vi "CalGas Filtern für Endpunktkalibrieren.vi"(10 "Messbereich":u16, 11 "CalGas":u16) -> (0 "Einheit":T4, 1 "Messberich":T4, 2 "Wert 2":T11 format="%#_5g", 3 "Wert 1":T11 format="%#_5g", 4 "Fehler":bool, 5 "Name":T4, 6 "Array":T1[](array[typedef]) format="%#_5g", 7 "Messbereich":u16)   [LabVIEW 2020, in "CalGas Aufschaltung.lvlib"]
uses:
  CalGas Aufschaltung.lvlib
  Visualisierungs Elemente/Zahlen-Ausgabefeld.ctl
  Visualisierungs Elemente/String - Ausgabefeld.ctl
  Definition CalGas Anzeige.ctl
  CalGas-Namen.ctl
  Visualisierungs Elemente/String - Eingabefeld.ctl
  CalGas-Werte.ctl
  Visualisierungs Elemente/Zahlen-Eingabefeld.ctl
  CalGas-Einheit.ctl
  Visualisierungs Elemente/Auswahlfeld.ctl
  CalGas-Messbereiche.ctl
  Aufschaltung CalGas_ANZEIGE.ctl
  FGV CalGas Aktionen.ctl
panel:
  in  "Aufschaltung CalGas":T2 {"Analysator" items=["FT-IR"]; "Aufschaltpunkt" items=["über Filterblock", "Analysator direkt", "über Gasteiler"]; "Kalibriergas" items=["Stickstoff", "", "", "", "", "", "", "", "", "", "", "", ""]}
  in  "Def.CalGas":T5 {"Messbereiche"."Messbereich 12" items=["0-100ppm", "0-1000ppm", "0-5000ppm"]; "Messbereiche"."Messbereich 11" items=["0-100ppm", "0-1000ppm", "0-5000ppm"]; "Messbereiche"."Messbereich 10" items=["0-100ppm", "0-1000ppm", "0-5000ppm"]; "Messbereiche"."Messbereich 9" items=["0-100ppm", "0-1000ppm", "0-5000ppm"]; "Messbereiche"."Messbereich 8" items=["0-100ppm", "0-1000ppm", "0-5000ppm"]; "Messbereiche"."Messbereich 7" items=["0-100ppm", "0-1000ppm", "0-5000ppm"]; "Messbereiche"."Messbereich 6" items=["0-100ppm", "0-1000ppm", "0-5000ppm"]; "Messbereiche"."Messbereich 5" items=["0-100ppm", "0-1000ppm", "0-5000ppm"]; "Messbereiche"."Messbereich 4" items=["0-100ppm", "0-1000ppm", "0-5000ppm"]; "Messbereiche"."Messbereich 3" items=["0-100ppm", "0-1000ppm", "0-5000ppm"]; "Messbereiche"."Messbereich 2" items=["0-100ppm", "0-1000ppm", "0-5000ppm"]; "Messbereiche"."Messbereich 1" items=["0-100ppm", "0-1000ppm", "0-5000ppm"]; "Einheit"."Einheit 12" items=["ppm", "%"]; "Einheit"."Einheit 11" items=["ppm", "%"]; "Einheit"."Einheit 10" items=["ppm", "%"]; "Einheit"."Einheit 9" items=["ppm", "%"]; "Einheit"."Einheit 8" items=["ppm", "%"]; "Einheit"."Einheit 7" items=["ppm", "%"]; "Einheit"."Einheit 6" items=["ppm", "%"]; "Einheit"."Einheit 5" items=["ppm", "%"]; "Einheit"."Einheit 4" items=["ppm", "%"]; "Einheit"."Einheit 3" items=["ppm", "%"]; "Einheit"."Einheit 2" items=["ppm", "%"]; "Einheit"."Einheit 1" items=["ppm", "%"]; "Werte 2"."Konzentration 12" format="%#_5g"; "Werte 2"."Konzentration 11" format="%#_5g"; "Werte 2"."Konzentration 10" format="%#_5g"; "Werte 2"."Konzentration 9" format="%#_5g"; "Werte 2"."Konzentration 8" format="%#_5g"; "Werte 2"."Konzentration 7" format="%#_5g"; "Werte 2"."Konzentration 6" format="%#_5g"; "Werte 2"."Konzentration 5" format="%#_5g"; "Werte 2"."Konzentration 4" format="%#_5g"; "Werte 2"."Konzentration 3" format="%#_5g"; "Werte 2"."Konzentration 2" format="%#_5g"; "Werte 2"."Konzentration 1" format="%#_5g"; "Werte"."Konzentration 12" format="%#_5g"; "Werte"."Konzentration 11" format="%#_5g"; "Werte"."Konzentration 10" format="%#_5g"; "Werte"."Konzentration 9" format="%#_5g"; "Werte"."Konzentration 8" format="%#_5g"; "Werte"."Konzentration 7" format="%#_5g"; "Werte"."Konzentration 6" format="%#_5g"; "Werte"."Konzentration 5" format="%#_5g"; "Werte"."Konzentration 4" format="%#_5g"; "Werte"."Konzentration 3" format="%#_5g"; "Werte"."Konzentration 2" format="%#_5g"; "Werte"."Konzentration 1" format="%#_5g"}
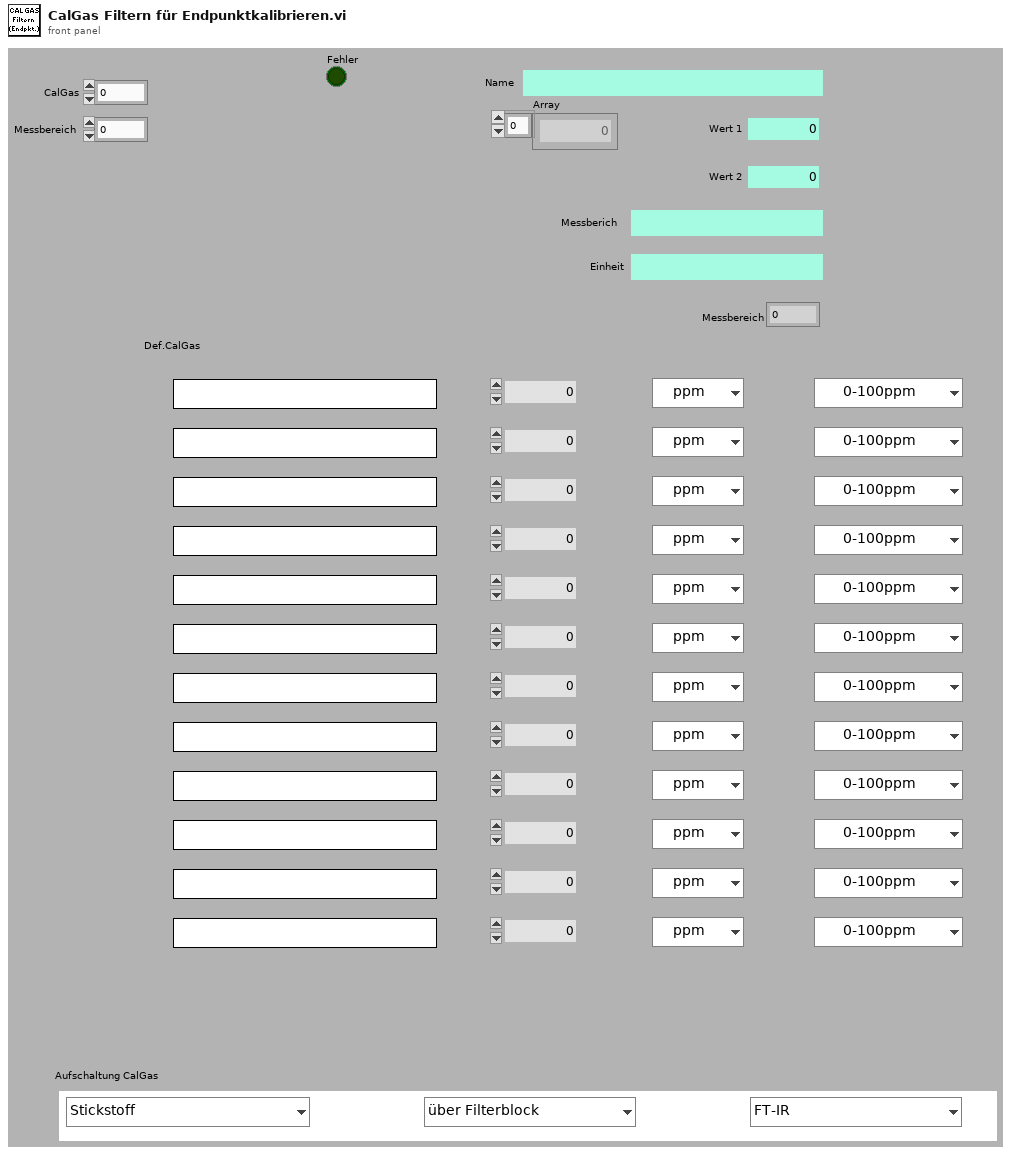
[diagram p1: front panel]
types:
  T1 = typedef "Zahlen-Eingabefeld.ctl" = sgl
  T2 = typedef "CalGas Aufschaltung.lvlib/Aufschaltung CalGas_ANZEIGE.ctl" = cluster{"Kalibriergas":T3, "Aufschaltpunkt":T3, "Analysator":T3}
  T3 = typedef "Auswahlfeld.ctl" = u16
  T4 = typedef "String - Ausgabefeld.ctl" = string
  T5 = typedef "CalGas Aufschaltung.lvlib/Definition CalGas Anzeige.ctl" = cluster{"Namen":T6, "Werte":T8, "Werte 2":T8, "Einheit":T9, "Messbereiche":T10}
  T6 = typedef "CalGas Aufschaltung.lvlib/CalGas-Namen.ctl" = cluster{"Name":T7, "Name 2":T7, "Name 3":T7, "Name 4":T7, "Name 5":T7, "Name 6":T7, "Name 7":T7, "Name 8":T7, "Name 9":T7, "Name 10":T7, "Name 11":T7, "Name 12":T7}
  T7 = typedef "String - Eingabefeld.ctl" = string
  T8 = typedef "CalGas Aufschaltung.lvlib/CalGas-Werte.ctl" = cluster{"Konzentration 1":T1, "Konzentration 2":T1, "Konzentration 3":T1, "Konzentration 4":T1, "Konzentration 5":T1, "Konzentration 6":T1, "Konzentration 7":T1, "Konzentration 8":T1, "Konzentration 9":T1, "Konzentration 10":T1, "Konzentration 11":T1, "Konzentration 12":T1}
  T9 = typedef "CalGas Aufschaltung.lvlib/CalGas-Einheit.ctl" = cluster{"Einheit 1":T3, "Einheit 2":T3, "Einheit 3":T3, "Einheit 4":T3, "Einheit 5":T3, "Einheit 6":T3, "Einheit 7":T3, "Einheit 8":T3, "Einheit 9":T3, "Einheit 10":T3, "Einheit 11":T3, "Einheit 12":T3}
  T10 = typedef "CalGas Aufschaltung.lvlib/CalGas-Messbereiche.ctl" = cluster{"Messbereich 1":T3, "Messbereich 2":T3, "Messbereich 3":T3, "Messbereich 4":T3, "Messbereich 5":T3, "Messbereich 6":T3, "Messbereich 7":T3, "Messbereich 8":T3, "Messbereich 9":T3, "Messbereich 10":T3, "Messbereich 11":T3, "Messbereich 12":T3}
  T11 = typedef "Zahlen-Ausgabefeld.ctl" = sgl
  T12 = typedef "CalGas Aufschaltung.lvlib/FGV CalGas Aktionen.ctl" = enum16{"lesen", "Analysator Auswahl", "Def.CalGas", "Aufschaltung CalGas", "laden", "speichern", "KAL extrahieren"}
  T13 = typedef "CalGas Aufschaltung.lvlib/Aufschaltung CalGas.ctl" = cluster{"Kalibriergas":T3, "Aufschaltpunkt":T14, "Analysator":T15}
  T14 = typedef "CalGas Aufschaltung.lvlib/Auswahl Aufschaltpunkt.ctl" = enum16{"über Filterblock", "Analysator direkt", "über PNS", "Entnahme", "Gasdivider"}
  T15 = typedef "CalGas Aufschaltung.lvlib/Auswahl Analysator.ctl" = enum16{"FT-IR", "FID", "PMA", "PMA/FID/FT-IR"}
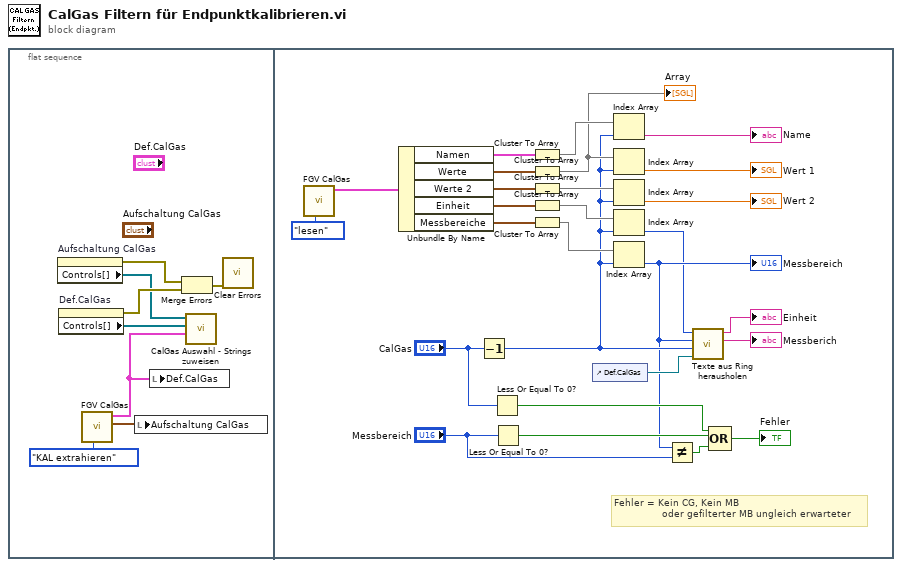
[diagram p0: block diagram]
diagram:
  n1 = flat-sequence {
    frame #0 {
      n2 = property on="Aufschaltung CalGas" class="Cluster (strikt)"() -> (error out=w8:errorcluster, "Controls[]"=w5:refnum<vi>[])  [unwired: 2 in, 1 out]
      n3 = property on="Def.CalGas" class="Cluster (strikt)"() -> (error out=w7:errorcluster, "Controls[]"=w6:refnum<vi>[])  [unwired: 2 in, 1 out]
      n4 = call "FGV CalGas.vi"("Aktionen"=FGV_CalGas_Aktionen."KAL extrahieren") -> ("Aufschaltung CalGas"=w4:T13, "Def.CalGas"=w1:T5)  [unwired: 6 in, 3 out]
      n5 = local write "Aufschaltung CalGas"(w4) -> ()
      n6 = local write "Def.CalGas"(w1) -> ()
      n7 = Merge Errors(w8, w7) -> (w2:errorcluster)
      n8 = call "CalGas Auswahl - Strings zuweisen.vi"(9:"Def.CalGas"=w1, 10:"Def.CalGas"=w6, "Aufschaltung CalGas"=w5) -> ()  [unwired: 8 in, 1 out]
      n9 = call <vilib>:"Clear Errors.vi"("error in (no error)"=w2) -> ()  [unwired: 5 in, 2 out]
    }
    frame #1 {
      # "Fehler = Kein CG, Kein MB\n                oder gefilterter MB ungleich erwarteter"
      n10 = call "FGV CalGas.vi"("Aktionen"=FGV_CalGas_Aktionen."lesen") -> ("Def.CalGas"=w24:T5)  [unwired: 6 in, 4 out]
      n11 = Unbundle By Name(w24) -> ("Namen"=w34:T6, "Werte"=w33:T8, "Werte 2"=w32:T8, "Einheit"=w31:T9, "Messbereiche"=w26:T10)
      n12 = Decrement(x="CalGas") -> (x-1=w16:u16)
      n13 = Less Or Equal To 0?(x="CalGas") -> (x <= 0?=w15:bool)
      n14 = Less Or Equal To 0?(x="Messbereich") -> (x <= 0?=w14:bool)
      n15 = Cluster To Array(cluster=w34) -> (array=w30:T7[])
      n16 = Cluster To Array(cluster=w33) -> (array=w29:T1[])
      "Array" <- w29
      n17 = Cluster To Array(cluster=w32) -> (array=w28:T1[])
      n18 = Cluster To Array(cluster=w31) -> (array=w27:T3[])
      n19 = Cluster To Array(cluster=w26) -> (array=w25:T3[])
      n20 = control-ref of="Def.CalGas"() -> (w23:refnum<vi>)
      n21 = Index Array(array=w30, index=w16) -> (element=→"Name":T7)
      n22 = Index Array(array=w29, index=w16) -> (element=→"Wert 1":T1)
      n23 = Index Array(array=w28, index=w16) -> (element=→"Wert 2":T1)
      n24 = Index Array(array=w27, index=w16) -> (element=w9:T3)
      n25 = Index Array(array=w25, index=w16) -> (element=w11:T3)
      "Messbereich" <- w11
      n26 = Not Equal?(x=w11, y="Messbereich") -> (x != y?=w13:bool)
      n27 = call "Texte aus Ring herausholen.vi"("Def.CalGas"=w23, "Gas"=w16, "Element Messbereich"=w11, "Element Einheit"=w9) -> ("Messberich"=→"Messberich":T4, "Einheit"=→"Einheit":T4)  [unwired: 6 in]
      n28 = Compound Arithmetic op=OR(w15, w14, w13) -> (→"Fehler":bool)
    }
  }
